vi "Time Diff Sub VI.vi"(1 "Start Time (hh:mm:ss)":string, 2 "Current Time (hh:mm:ss)":string) -> (0 "Time Diff (s)":i32)   [LabVIEW 2015]
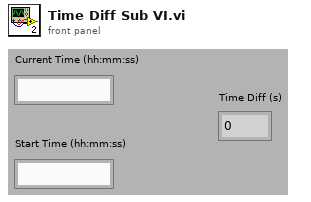
[diagram p1: front panel]
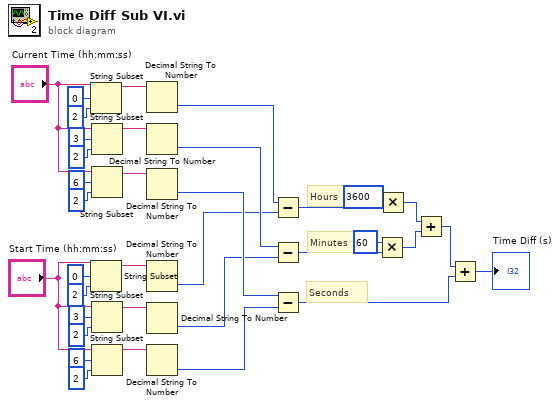
[diagram p0: block diagram]
diagram:
  # "Seconds"
  # "Minutes"
  # "Hours"
  n1 = String Subset(string="Current Time (hh:mm:ss)", offset (0)=0, length (rest)=2 ("length (rest)")) -> (substring=w21:string)
  n2 = String Subset(string="Start Time (hh:mm:ss)", offset (0)=0, length (rest)=2 ("length (rest)")) -> (substring=w18:string)
  n3 = String Subset(string="Current Time (hh:mm:ss)", offset (0)=3, length (rest)=2 ("length (rest)")) -> (substring=w20:string)
  n4 = String Subset(string="Current Time (hh:mm:ss)", offset (0)=6, length (rest)=2 ("length (rest)")) -> (substring=w19:string)
  n5 = String Subset(string="Start Time (hh:mm:ss)", offset (0)=3, length (rest)=2 ("length (rest)")) -> (substring=w17:string)
  n6 = String Subset(string="Start Time (hh:mm:ss)", offset (0)=6, length (rest)=2 ("length (rest)")) -> (substring=w16:string)
  n7 = Decimal String To Number(string=w21) -> (number=w15:i32)  [unwired: 3 out]
  n8 = Decimal String To Number(string=w20) -> (number=w14:i32)  [unwired: 3 out]
  n9 = Decimal String To Number(string=w19) -> (number=w13:i32)  [unwired: 3 out]
  n10 = Decimal String To Number(string=w18) -> (number=w1:i32)  [unwired: 3 out]
  n11 = Decimal String To Number(string=w17) -> (number=w2:i32)  [unwired: 3 out]
  n12 = Decimal String To Number(string=w16) -> (number=w12:i32)  [unwired: 3 out]
  n13 = Subtract(x=w15, y=w1) -> (x-y=w11:i32)
  n14 = Subtract(x=w14, y=w2) -> (x-y=w10:i32)
  n15 = Subtract(x=w13, y=w12) -> (x-y=w4:i32)
  n16 = Multiply(x=60, y=w10) -> (x*y=w7:i32)
  n17 = Multiply(x=3600, y=w11) -> (x*y=w6:i32)
  n18 = Add(x=w6, y=w7) -> (x+y=w5:i32)
  n19 = Add(x=w5, y=w4) -> (x+y=→"Time Diff (s)":i32)
